vi "im_to_array_lfTester.vi"(1 "Optional Rectangle":i32[](array[numeric])=[100, 1131, 386, 1303], 2 "Image file path":path) -> (0 "Pixels Values":u8[][](array[numeric]))   [LabVIEW 2017]
doc: "This example shows how to convert an image into a two-dimensional LabVIEW array. By converting an image into a LabVIEW array, you can apply all the analysis, display, and array operators available in LabVIEW to the image data."
panel:
  out "Image Source":T1(plugin-control)
  # "Overview: Demonstrates how to retrieve an array of pixel values from an image.\nRequirements: NI Vision Development Module\nInstructions: Run the VI."
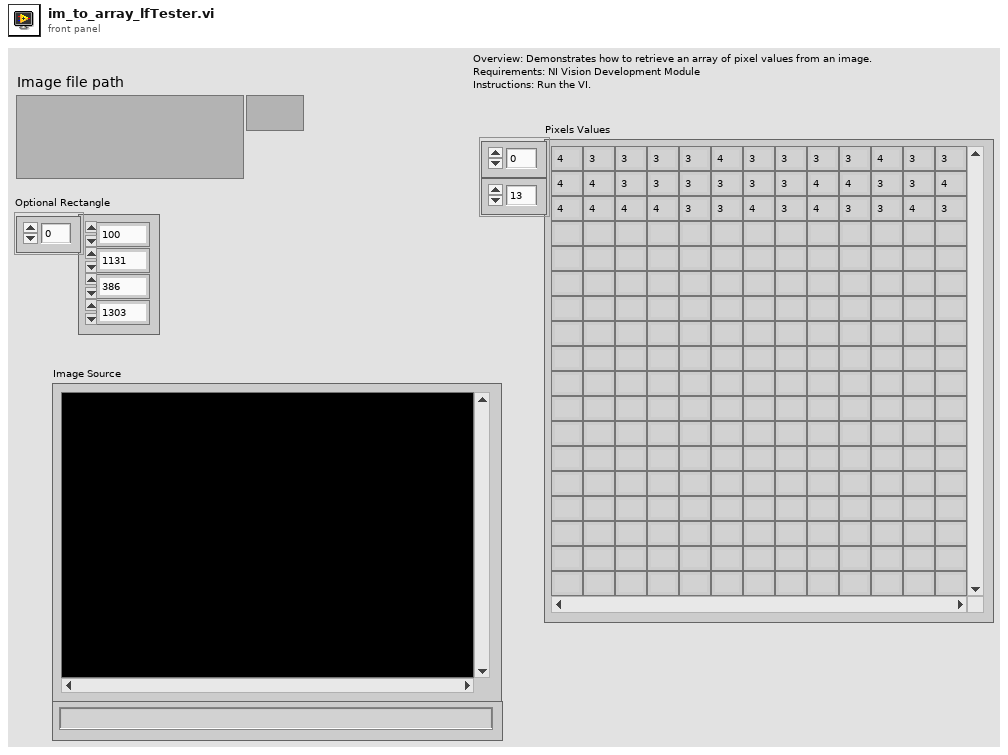
[diagram p1: front panel]
types:
  T1 = typedef "IMAQ Image.ctl" = refnum<image>
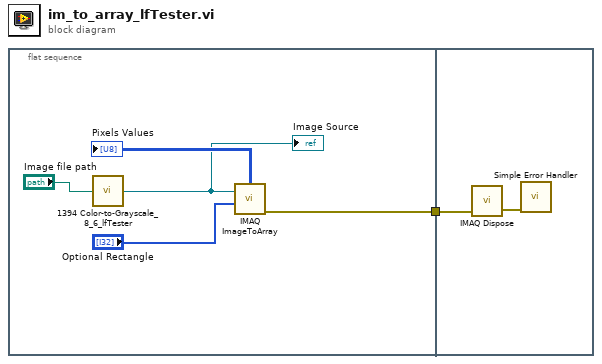
[diagram p0: block diagram]
diagram:
  n1 = flat-sequence {
    tunnel: [w5] -> w1
    tunnel: w1 -> [w7]
    frame #0 {
      n2 = call "1394 Color-to-Grayscale_8_6_lfTester.vi"("File Path"="Image file path") -> ("Luminance Plane"=w2:T1)
      "Image Source" <- w2
      n3 = call "IMAQ ImageToArray"("Optional Rectangle"="Optional Rectangle", "Image"=w2) -> ("error out"=w5:errorcluster, "Image Pixels (U8)"=→"Pixels Values":u8[][])  [unwired: 2 in, 3 out]
    }
    frame #1 {
      n4 = call "IMAQ Dispose"("error in (no error)"=w7) -> ("error out"=w8:errorcluster)  [unwired: 5 in]
      n5 = call <vilib>:"Simple Error Handler.vi"("error in (no error)"=w8) -> ()  [unwired: 4 in, 5 out]
    }
  }
